vi "TestVI_Spectrometer.vi"() -> ()   [LabVIEW 2018]
panel:
  in  "Independent?":bool=TRUE
  in  "File Close Action":enum16{"Prompt", "Keep", "Archive", "Trash"}(ring)
  out "VI name":string="TestVI_Spectrometer"
  out "file path":path=path "C:/Users/aspit/Git/MHDLab/Test Data/2018-06-02/H2TC/Temp Dependence/TestVI_Spectrometer_200C.tdms"
  in  "File Information":T1={"Project"=enum."H2TC", "SubFolder"="Temp Dependence", "Filename (Meas. Description)"="200C", "Measurement number"=0}
  out "tdms error":errorcluster
  out "tdms file":refnum<k34>
  out "output cluster":cluster{"Sine with Uniform Noise":dynamicdata}={"Sine with Uniform Noise"=[{"t0"=timestamp(3610818365.639246 s since 1904-01-01), "dt"=0.001, "Y"=[0.7822705518004847], "attributes"=variant("NI_ChannelName"=variant(string "Sine with Uniform Noise"), "NI_ExpIsRelativeTime"=variant(bool FALSE), "NI_ExpStartTimeStamp"=variant(timestamp timestamp(3610818355.905246 s since 1904-01-01)), "NI_ExpTimeStamp"=variant(timestamp timestamp(3610818365.639246 s since 1904-01-01)), "NI_ExpXDimension"=variant(string "t"))}]}
  out "Sine with Uniform Noise":dbl=0.7822705518004847
  in  "stop":bool
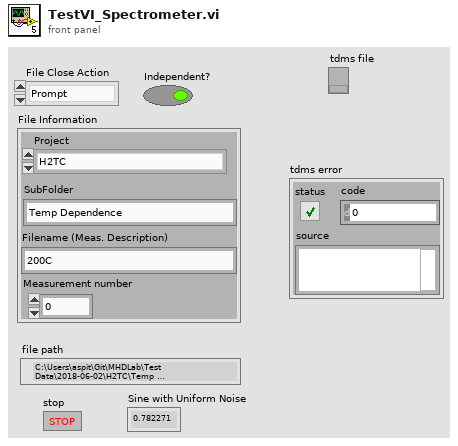
[diagram p1: front panel]
types:
  T1 = cluster{"Project":enum16{"H2TC", "VAPOR1"}, "SubFolder":string, "Filename (Meas. Description)":string, "Measurement number":i32}
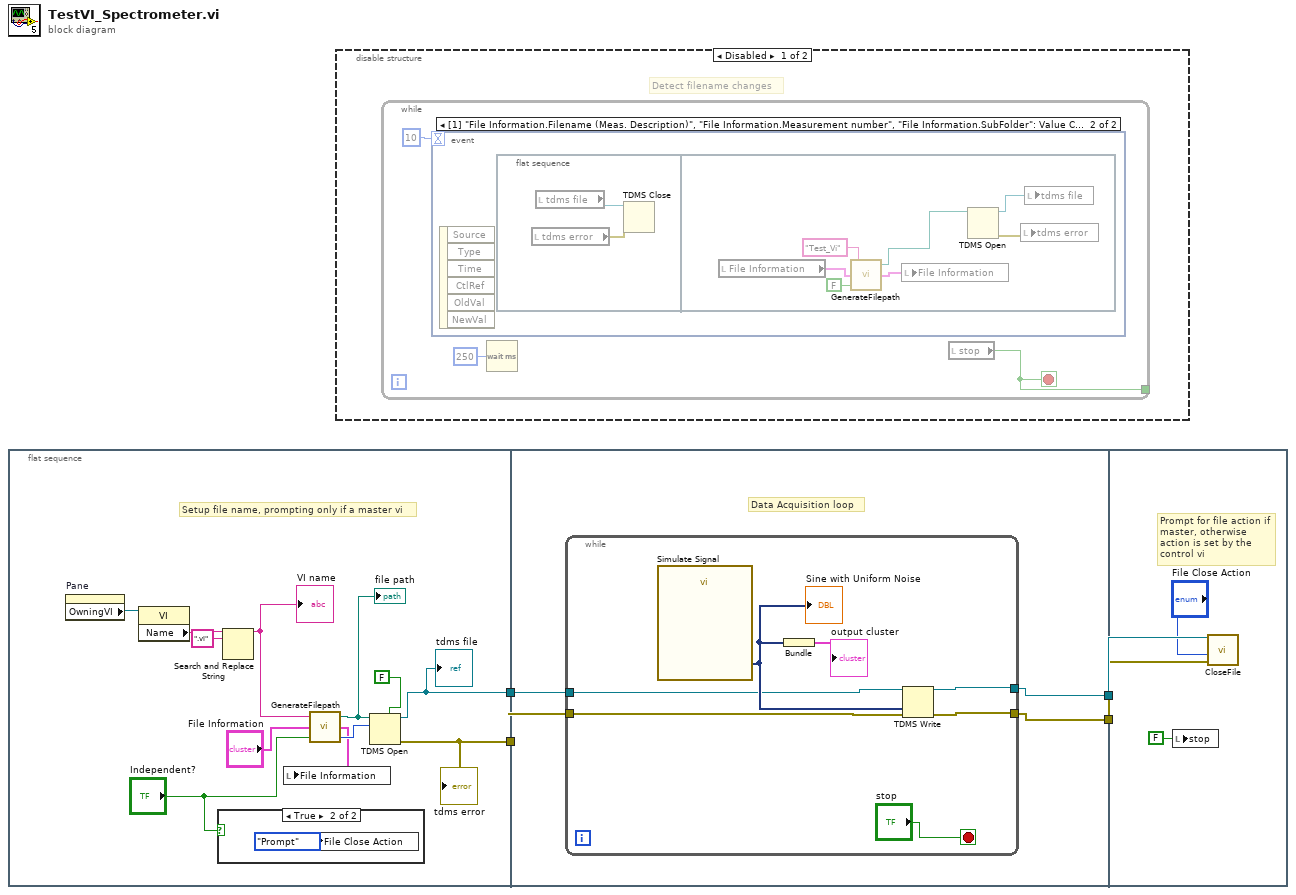
[diagram p0: block diagram]
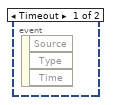
[diagram p3: hidden frame]
diagram:
  n1 = flat-sequence {
    tunnel: [w9] -> w4
    tunnel: [w8] -> w3
    tunnel: w4 -> [w21]
    tunnel: w3 -> [w20]
    tunnel: [w19] -> w2
    tunnel: [w18] -> w1
    tunnel: w2 -> [w31]
    tunnel: w1 -> [w32]
    frame #0 {
      # "Setup file name, prompting only if a master vi"
      n2 = property on="Pane" class="Pane"() -> ("OwningVI"=w15:refnum<vi>)  [unwired: 2 in, 2 out]
      n3 = property class="VI"(reference=w15) -> ("Name"=w16:string)  [unwired: 1 in, 2 out]
      n4 = case shown="True" "Independent?" {
        frame False {
        }
        frame True {
          n5 = local write "File Close Action"(enum16{"Prompt", "Keep", "Archive", "Trash"}."Prompt" ("File Close Action")) -> ()
        }
      }
      n6 = Search and Replace String(input string=w16, search string=".vi") -> (result string=w7:string)  [unwired: 6 in, 3 out]
      "VI name" <- w7
      n7 = call "GenerateFilepath.vi"("Check for file?"="Independent?", "File Information"="File Information", "Instrument"=w7) -> ("File Action"=w13:i32, "File Information Out"=w12:T1, "File Path Out"=w6:path)
      "file path" <- w6
      n8 = local write "File Information"(w12) -> ()
      n9 = TDMS Open(5:FALSE ("create index file? (T)"), 10:w13, 11:w6) -> (0:w9:errorcluster, 3:w8:refnum<k34>)  [unwired: 4 in]
      "tdms file" <- w8
      "tdms error" <- w9
    }
    frame #1 {
      # "Data Acquisition loop"
      n10 = while {
        tunnel: [w25] -> w18
        tunnel: [w24] -> w19
        tunnel: w21 -> [w23]
        tunnel: w20 -> [w22]
        stop <- "stop" stop-if-true
        n11 = call "Simulate Signal"() -> ("Sine with Uniform Noise"=w26:dynamicdata)  [unwired: 14 in, 1 out]
        "Sine with Uniform Noise" <- w26
        n12 = Bundle("Sine with Uniform Noise"=w26) -> (→"output cluster":cluster{"Sine with Uniform Noise":dynamicdata})  [unwired: 1 in]
        n13 = TDMS Write(0:w22, 9:w26, 11:w23) -> (4:w25:refnum<k34>, 15:w24:errorcluster)  [unwired: 3 in, 2 out]
      }
    }
    frame #2 {
      # "Prompt for file action if master, otherwise action is set by the control vi"
      n14 = local write "stop"(FALSE ("stop")) -> ()
      n15 = call "CloseFile.vi"("error in (no error)"=w31, "Action"="File Close Action", "Refnum in"=w32) -> ()  [unwired: 8 in, 1 out]
    }
  }
  n16 = disable-structure shown="Disabled" {
    frame Disabled {
      # "Detect filename changes"
      n17 = while {
        tunnel: [w33] -> _
        stop <- w33 stop-if-true
        n18 = event shown="[1] \"File Information.Filename (Meas. Description)\", \"File Information.Measurement number\", \"File Information.SubFolder\": Value Change" {
          selector: _ -> [_ _]
          dyn-events: _ -> [_ _]
          timeout: 10 -> [_ _]
          event Timeout {
            n19 = event-data() -> ()  [unwired: 1 in, 3 out]
          }
          event "File Information.Filename (Meas. Description)", "File Information.Measurement number", "File Information.SubFolder": Value Change {
            n20 = event-data() -> ()  [unwired: 1 in, 6 out]
            n21 = flat-sequence {
              frame #0 {
                n22 = local read "tdms error"() -> (w37:errorcluster)
                n23 = local read "tdms file"() -> (w36:refnum<k34>)
                n24 = TDMS Close(8:w37, 11:w36) -> ()  [unwired: 2 out]
              }
              frame #1 {
                n25 = local read "File Information"() -> (w42:T1)
                n26 = call "GenerateFilepath.vi"("Check for file?"=FALSE, "File Information"=w42, "Instrument"="Test_Vi") -> ("File Information Out"=w44:T1, "File Path Out"=w41:path)  [unwired: 1 out]
                n27 = local write "File Information"(w44) -> ()
                n28 = TDMS Open(11:w41) -> (0:w39:errorcluster, 3:w40:refnum<k34>)  [unwired: 6 in]
                n29 = local write "tdms error"(w39) -> ()
                n30 = local write "tdms file"(w40) -> ()
              }
            }
          }
        }
        n31 = Wait (ms)(milliseconds to wait=u32 250) -> ()  [unwired: 1 out]
        n32 = local read "stop"() -> (w33:bool)
      }
    }
    frame Enabled {
    }
  }
